vi "Move To Abs sw.vi"(8 "error in (no error)":errorcluster, 9 "Step In range":bool, 10 "Possition selector":T1(radio), 11 "Lifter_motor in":refnum<class "Lifter_motor.lvclass">) -> (0 "error out":errorcluster, 3 "Lifter_motor out":refnum<class "Lifter_motor.lvclass">)   [LabVIEW 2019, in "Lifter_motor.lvclass"]
uses:
  Lifter_motor.lvclass
  Lifter_motor.lvclass/Lifter_motor.ctl
panel:
  out "Driver ACK?":bool
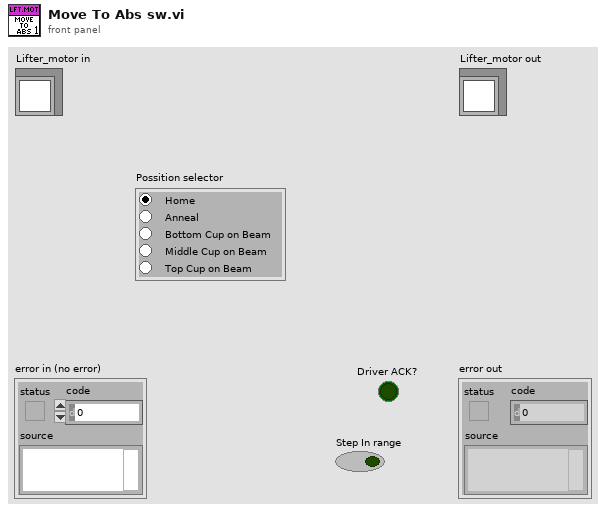
[diagram p1: front panel]
types:
  T1 = enum32{"Home", "Anneal", "Bottom Cup on Beam", "Middle Cup on Beam", "Top Cup on Beam"}
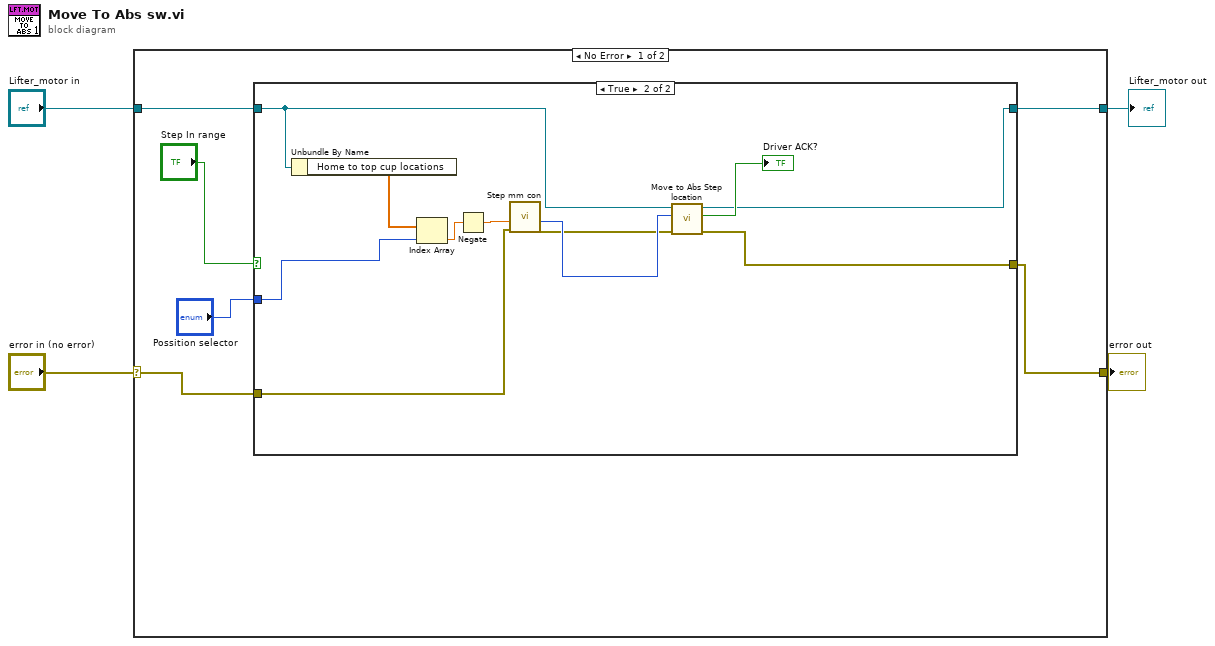
[diagram p0: block diagram]
diagram:
  n1 = case shown="No Error" "error in (no error)" {
    selector: "error in (no error)" -> [w7 w25]
    tunnel: [w6 w25] -> w3
    tunnel: "Lifter_motor in" -> [w9 w24]
    tunnel: [w8 w24] -> w1
    frame No Error {
      n2 = case shown="True" "Step In range" {
        tunnel: "Possition selector" -> [_ w23]
        tunnel: w9 -> [w12 w13]
        tunnel: [w12 w18] -> w8
        tunnel: w7 -> [w11 w16]
        tunnel: [w11 w17] -> w6
        frame False {
        }
        frame True {
          n3 = Unbundle By Name(w13) -> ("Home to top cup locations"=w20:dbl[])
          n4 = Index Array(array=w20, index=w23) -> (element=w21:dbl)
          n5 = Negate(x=w21) -> (-x=w22:dbl)
          n6 = call "Step mm con.vi"("error in (no error)"=w16, "mm in"=w22) -> ("error out"=w14:errorcluster, "step out"=w15:i32)  [unwired: 7 in, 1 out]
          n7 = call "Move to Abs Step location.vi"("error in (no error)"=w14, "Absolute step location to move"=w15, "Lifter_motor in"=w13) -> ("error out"=w17:errorcluster, "Driver ACK?"=→"Driver ACK?":bool, "Lifter_motor out"=w18:refnum<class "Lifter_motor.lvclass">)  [unwired: 6 in]
        }
      }
    }
    frame Error {
    }
  }
  "error out" <- w3
  "Lifter_motor out" <- w1
